vi "Item_OnPopupMenu.vi"(11 "Object":T1) -> ()   [LabVIEW 2020, in "Project Provider.lvlib"]
uses:
  Project Provider.lvlib
  <resource>/Framework/Providers/API/ItemRef.ctl
  <resource>/Framework/Providers/API/mxLvMenuItem.ctl
panel:
  out "error out":errorcluster
  in  "error in":errorcluster
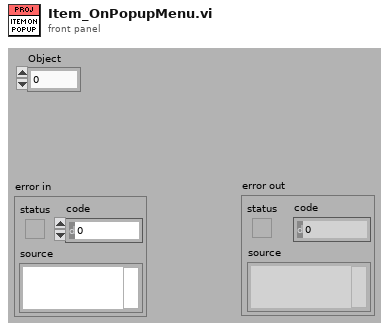
[diagram p1: front panel]
types:
  T1 = typedef "ItemRef.ctl" = u64
  T2 = typedef "mxLvMenuItem.ctl" = cluster{"Menu Name":string, "Description":string, "Icon File Name":path, "Menu Tag":string, "Enabled":bool, "Checked":bool, "Separator":bool, "Batchable":bool, "Weight":i32, "Batch Mode (Ignored if Not Batchable)":enum32{"Show If All Items Support Command", "Show If Any Items Support Command"}, "Menu Location":enum32{"<None>", "Project", "Project / Build Specifications", "Tools", "Tools / Source Control", "Tools / Real-Time Module", "Help"}, "Exclude From Getting Started Window Menu":bool}
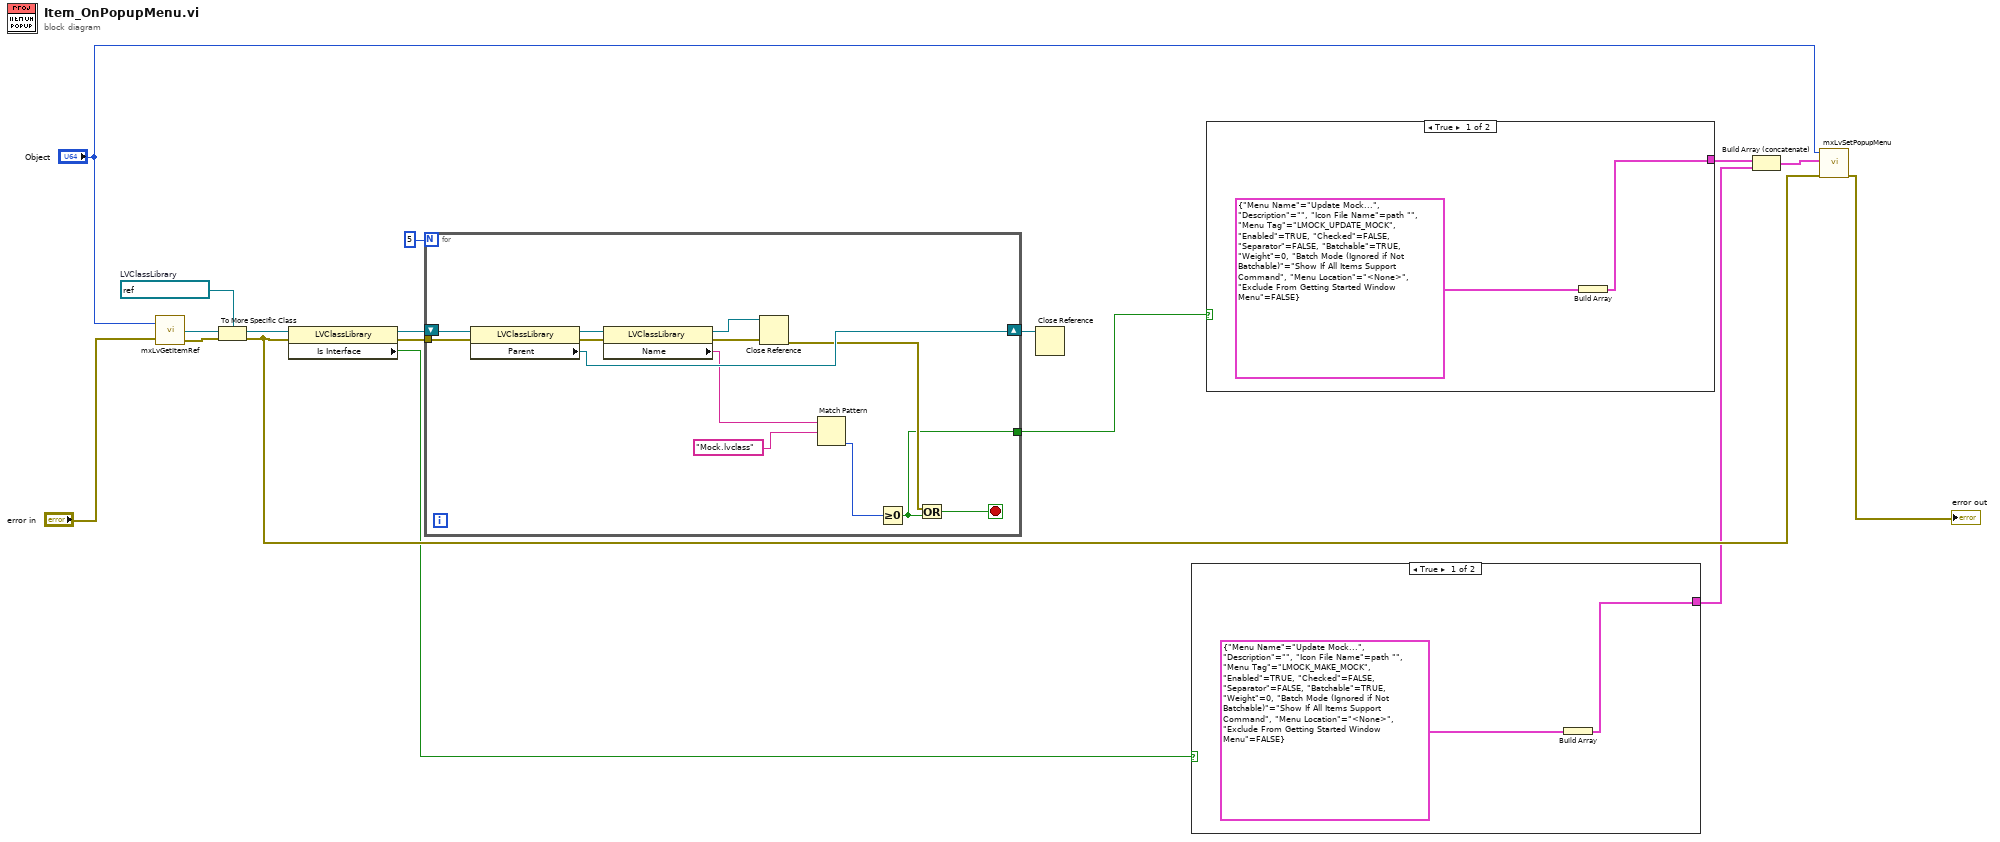
[diagram p0: block diagram]
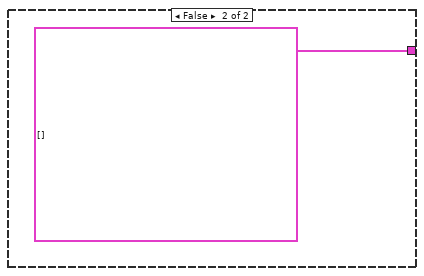
[diagram p2: hidden frame]
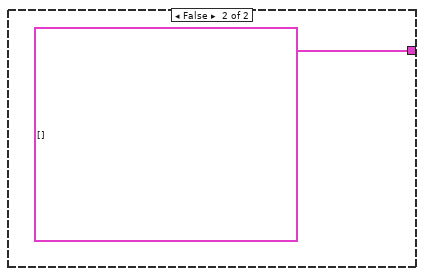
[diagram p3: hidden frame]
diagram:
  w16 = refnum<vi> refnum  # LVClassLibrary
  n1 = call <resource>:"mxLvGetItemRef.vi"("Item"="Object", "error in"="error in") -> ("Item Refnum"=w17:refnum<vi>, "error out"=w15:errorcluster)  [unwired: 1 out]
  n2 = To More Specific Class(target class=w16, reference=w17, error in=w15) -> (specific class reference=w5:refnum<vi>, error out=w3:errorcluster)
  n3 = property class="LVClassLibrary"(reference=w5, error in=w3) -> (reference out=w4:refnum<vi>, error out=w6:errorcluster, "Is Interface"=w1:bool)
  n4 = for {
    N: 5 -> [_]
    tunnel: w6 -> [w29]
    shift-right: [w28] -> w12
    shift-left: w4 -> [w30]
    tunnel: [w18] -> w10
    stop <- w20 stop-if-true
    n5 = property class="LVClassLibrary"(reference=w30, error in=w29) -> (reference out=w25:refnum<vi>, error out=w23:errorcluster, "Parent"=w28:refnum<vi>)
    n6 = property class="LVClassLibrary"(reference=w25, error in=w23) -> (reference out=w24:refnum<vi>, error out=w22:errorcluster, "Name"=w27:string)
    n7 = Close Reference(reference=w24, error in (no error)=w22) -> (error out=w26:errorcluster)
    n8 = Match Pattern(string=w27, regular expression="Mock.lvclass" ("element")) -> (offset past match=w19:i32)  [unwired: 1 in, 3 out]
    n9 = Greater Or Equal To 0?(x=w19) -> (x >= 0?=w18:bool)
    n10 = Or(x=w26, y=w18) -> (x .or. y?=w20:bool)
  }
  n11 = Close Reference(reference=w12) -> ()  [unwired: 1 in, 1 out]
  n12 = case shown="True" w1 {
    tunnel: [w31 T2[] []] -> w2
    frame True {
      n13 = Build Array(T2 {"Menu Name"="Update Mock...", "Description"="", "Icon File Name"=path "", "Menu Tag"="LMOCK_MAKE_MOCK", "Enabled"=TRUE, "Checked"=FALSE, "Separator"=FALSE, "Batchable"=TRUE, "Weight"=0, "Batch Mode (Ignored if Not Batchable)"=enum."Show If All Items Support Command", "Menu Location"=enum."<None>", "Exclude From Getting Started Window Menu"=FALSE} ("Menu Item")) -> (w31:T2[])
    }
    frame False {
    }
  }
  n14 = case shown="True" w10 {
    tunnel: [w34 T2[] []] -> w9
    frame True {
      n15 = Build Array(T2 {"Menu Name"="Update Mock...", "Description"="", "Icon File Name"=path "", "Menu Tag"="LMOCK_UPDATE_MOCK", "Enabled"=TRUE, "Checked"=FALSE, "Separator"=FALSE, "Batchable"=TRUE, "Weight"=0, "Batch Mode (Ignored if Not Batchable)"=enum."Show If All Items Support Command", "Menu Location"=enum."<None>", "Exclude From Getting Started Window Menu"=FALSE} ("Menu Item")) -> (w34:T2[])
    }
    frame False {
    }
  }
  n16 = Build Array (concatenate)(w9, w2) -> (w7:T2[])
  n17 = call <resource>:"mxLvSetPopupMenu.vi"("error in"=w3, "Popup Menu Items"=w7, "Item"="Object") -> ("error out"=→"error out":errorcluster)  [unwired: 7 in, 1 out]
